vi "ImageListManager.vi"(8 "filename":string, 10 "Header Title String":string="Image List", 11 "Image Information In":T1) -> (3 "Image Information Out":T1)   [LabVIEW 2013]
uses:
  ImageInfoList.ctl
  <vilib>/Utility/sysdir.llb/System Directory Type.ctl
  <vilib>/Utility/xml.llb/Write to XML File(string).vi
  <vilib>/Utility/xml.llb/Read From XML File(string).vi
panel:
  out "Boolean References":refnum<vi>[](array[refnum])
  in  "Tab Control":enum32{"List", "Add"}(tab)
  in  "Image List":i32(listbox)
  in  "Add Button":bool
  in  "Remove Button":bool
  in  "Image Frequency (seconds)":dbl=30.0 min=30.0 step=1.0
  in  "Save Button":bool
  in  "Load Button":bool
  in  "Cancel Button":bool
  in  "OK Button":bool
  out "Help":string="This is the image management utility. \n\nTo add an image to the image list, click \"Add Image\" and you will be taken to the Add Image screen.  Provide a \"helpful name\" for the image either enter a file path to the image file or use the folder icon to browse.  You will be given a preview of your file.  To add the file to the list, press NEXT.  To exit the screen, press BACK.\n\nTo remove an image, select the image in the list and press \"Remove Image\".\n\nTo save your list of images, click \"Save List\".  To load your list of images for edit, click \"Load List\".  Lists will be saved in XML format.  Please do not edit the XML files directly.\n\nTo select the image frequency - or the amount of time between image updates, enter the Image Frequency into the box marked, \"Image Frequency (seconds)\".  \n\nTo accept this list of images, press OK.  To cancel all changes, press CANCEL."
  out "Error Messages":errorcluster
  out "Image Preview":picture
  in  "Back Button":bool
  in  "Next Button":bool
  in  "Image Path":path
  out "Add Image String":string="Add New Image"
  in  "Image Nickname":string
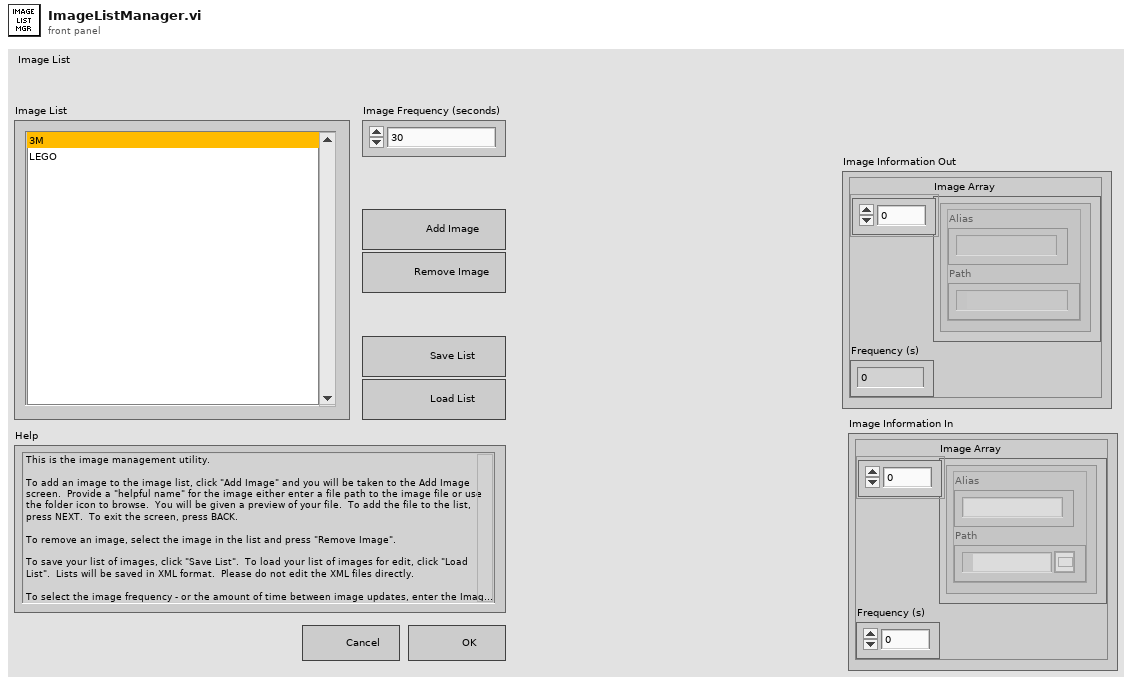
[diagram p1: front panel]
types:
  T1 = typedef "ImageInfoList.ctl" = cluster{"Image Array":cluster{"Alias":string, "Path":path}[], "Frequency (s)":dbl}
  T2 = enum8{"Enabled", "Disabled", "Disabled and Grayed Out"}
  T3 = typedef "System Directory Type.ctl" = i32
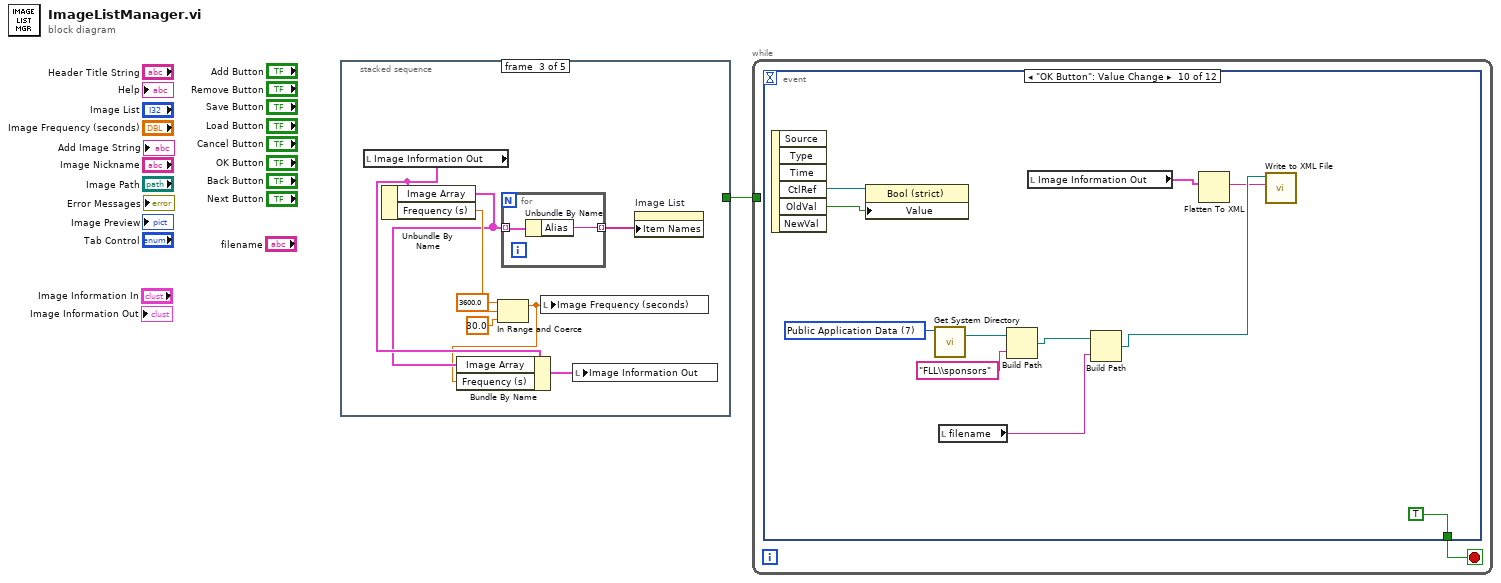
[diagram p0: block diagram]
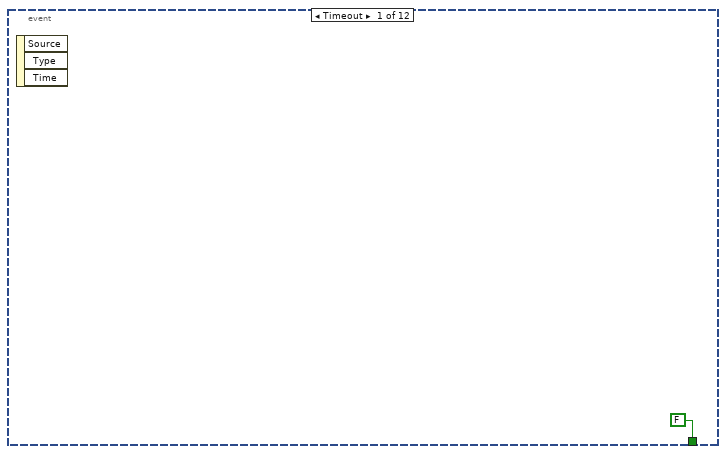
[diagram p2: hidden frame]
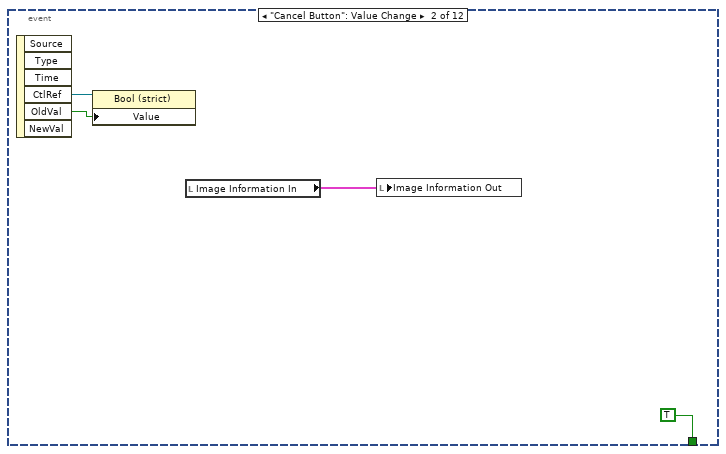
[diagram p3: hidden frame]
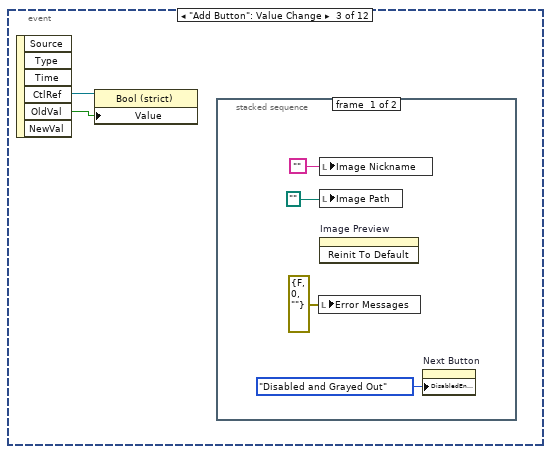
[diagram p4: hidden frame]
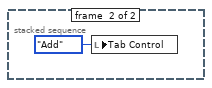
[diagram p5: hidden frame]
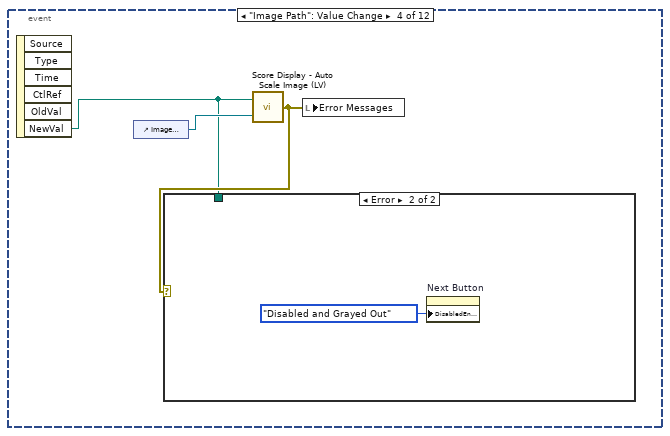
[diagram p6: hidden frame]
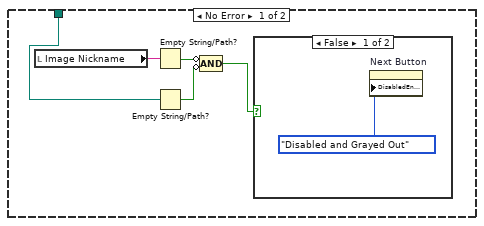
[diagram p7: hidden frame]
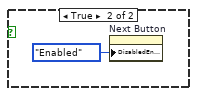
[diagram p8: hidden frame]
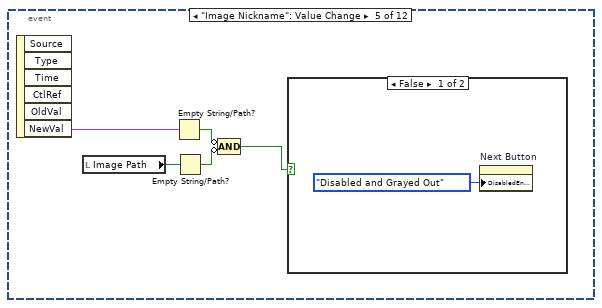
[diagram p9: hidden frame]
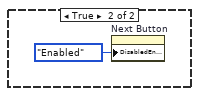
[diagram p10: hidden frame]
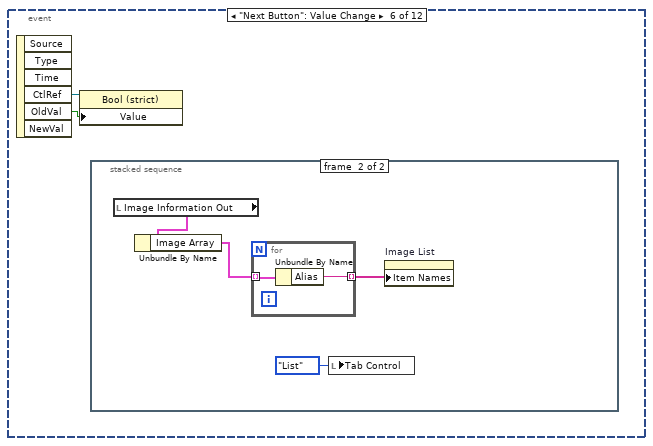
[diagram p11: hidden frame]
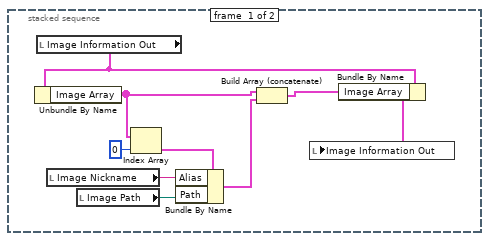
[diagram p12: hidden frame]
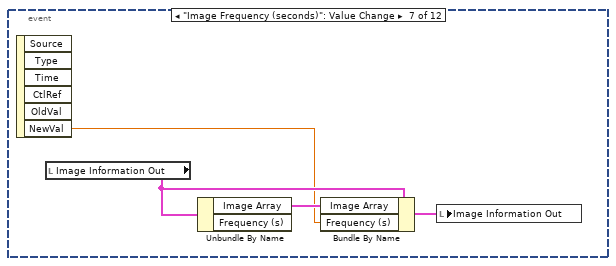
[diagram p13: hidden frame]
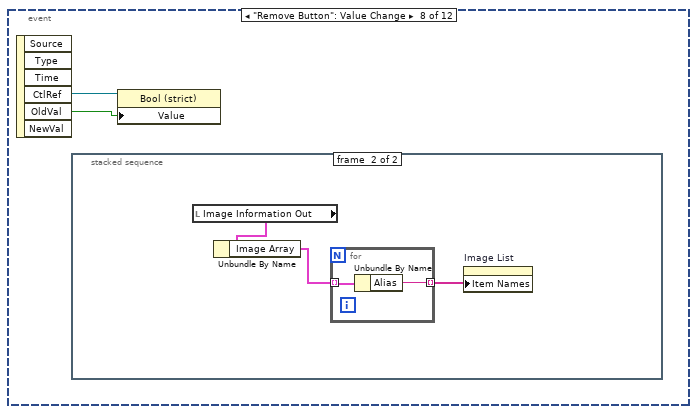
[diagram p14: hidden frame]
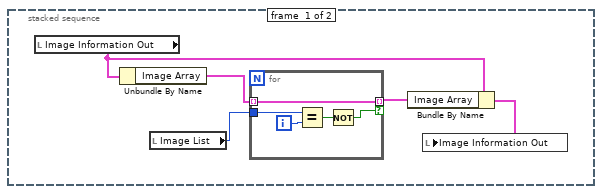
[diagram p15: hidden frame]
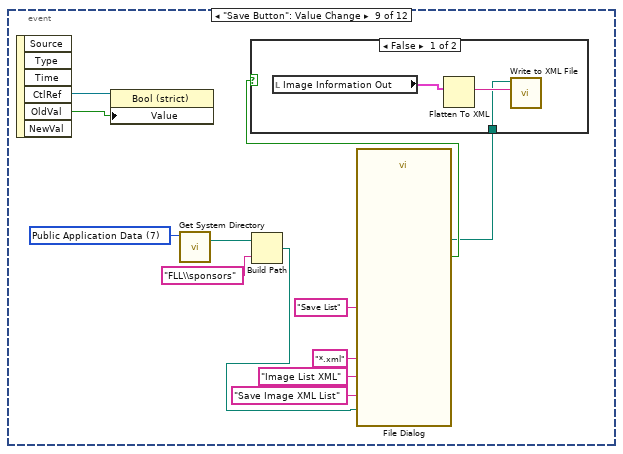
[diagram p16: hidden frame]
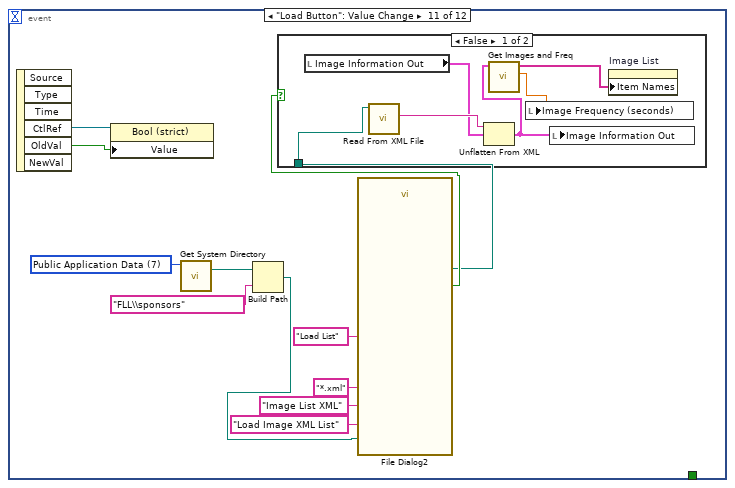
[diagram p18: hidden frame]
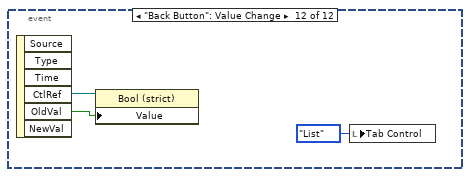
[diagram p20: hidden frame]
diagram:
  n1 = stacked-sequence {
    tunnel: [_ _ _ _ FALSE] -> w1
    frame #0 {
      n2 = control-ref of="Add Button"() -> (w2:refnum<vi>)
      n3 = control-ref of="Remove Button"() -> (w3:refnum<vi>)
      n4 = control-ref of="Save Button"() -> (w4:refnum<vi>)
      n5 = control-ref of="Load Button"() -> (w5:refnum<vi>)
      n6 = control-ref of="Cancel Button"() -> (w6:refnum<vi>)
      n7 = control-ref of="OK Button"() -> (w7:refnum<vi>)
      n8 = control-ref of="Back Button"() -> (w8:refnum<vi>)
      n9 = control-ref of="Next Button"() -> (w9:refnum<vi>)
      n10 = Build Array(w2, w3, w4, w5, w6, w7, w8, w9) -> (→"Boolean References":refnum<vi>[])
    }
    frame #1 {
      n11 = local read "Image Information In"() -> (w12:T1)
      n12 = local write "Tab Control"(enum32{"List", "Add"}."List" ("Tab Control")) -> ()
      n13 = local write "Image Information Out"(w12) -> ()
    }
    frame #2 {
      n14 = local read "Image Information Out"() -> (w15:T1)
      n15 = Unbundle By Name(w15) -> ("Image Array"=w14:cluster{"Alias":string, "Path":path}[], "Frequency (s)"=w19:dbl)
      n16 = In Range and Coerce(upper limit=3600.0, x=w19, lower limit=30.0) -> (coerced(x)=w13:dbl)  [unwired: 1 out]
      n17 = Bundle By Name(cluster=w15, "Image Array"=w14, "Frequency (s)"=w13) -> (w16:T1)
      n18 = for {
        tunnel: w14 -> [w22] mode=indexing
        tunnel: [w21] -> w20 mode=indexing
        n19 = Unbundle By Name(w22) -> ("Alias"=w21:string)
      }
      n20 = local write "Image Frequency (seconds)"(w13) -> ()
      n21 = local write "Image Information Out"(w16) -> ()
      n22 = property on="Image List" class="LstBox (strict)"("Item Names"=w20) -> ()  [unwired: 2 in, 2 out]
    }
    frame #3 {
      # "Initialize - Set Booleans to False"
      n23 = local read "Boolean References"() -> (w23:refnum<vi>[])
      n24 = for {
        tunnel: w23 -> [w25] mode=indexing
        n25 = property class="Bool (strict)"(reference=w25, "Value"=FALSE) -> ()  [unwired: 1 in, 2 out]
      }
    }
    frame #4 {
    }
  }
  n26 = while {
    tunnel: w1 -> [_]
    stop <- w27 stop-if-true
    n27 = event shown="[9] \"OK Button\": Value Change" {
      selector: _ -> [_ _ _ _ _ _ _ _ _ _ _ _]
      dyn-events: _ -> [_ _ _ _ _ _ _ _ _ _ _ _]
      timeout: _ -> [_ _ _ _ _ _ _ _ _ _ _ _]
      tunnel: [FALSE TRUE _ _ _ _ _ _ _ TRUE _ _] -> w27
      event Timeout {
        n28 = event-data() -> ()  [unwired: 1 in, 3 out]
      }
      event "Cancel Button": Value Change {
        n29 = event-data() -> ("CtlRef"=w30:refnum<vi>, "OldVal"=w29:bool)  [unwired: 1 in, 4 out]
        n30 = property class="Bool (strict)"(reference=w30, "Value"=w29) -> ()  [unwired: 1 in, 2 out]
        n31 = local read "Image Information In"() -> (w32:T1)
        n32 = local write "Image Information Out"(w32) -> ()
      }
      event "Add Button": Value Change {
        n33 = event-data() -> ("CtlRef"=w34:refnum<vi>, "OldVal"=w33:bool)  [unwired: 1 in, 4 out]
        n34 = property class="Bool (strict)"(reference=w34, "Value"=w33) -> ()  [unwired: 1 in, 2 out]
        n35 = stacked-sequence {
          frame #0 {
            n36 = local write "Error Messages"(errorcluster {"status"=FALSE, "code"=0, "source"=""} ("Error Messages")) -> ()
            n37 = local write "Image Nickname"("") -> ()
            n38 = local write "Image Path"(path "") -> ()
            n39 = invoke on="Image Preview" class="Pict" method="Reinit To Default"() -> ()  [unwired: 3 in, 3 out]
            n40 = property on="Next Button" class="Bool (strict)"("DisabledEnum"=T2."Disabled and Grayed Out" ("Disabled")) -> ()  [unwired: 2 in, 2 out]
          }
          frame #1 {
            n41 = local write "Tab Control"(enum32{"List", "Add"}."Add" ("Tab Control")) -> ()
          }
        }
      }
      event "Image Path": Value Change {
        n42 = event-data() -> ("NewVal"=w40:path)  [unwired: 1 in, 5 out]
        n43 = control-ref of="Image Preview"() -> (w42:refnum<vi>)
        n44 = call "Score Display - Auto Scale Image (LV).vi"("Picture Reference"=w42, "path to image file"=w40) -> ("error out"=w41:errorcluster)
        n45 = case shown="Error" w41 {
          tunnel: w40 -> [w45 _]
          frame No Error {
            n46 = local read "Image Nickname"() -> (w47:string)
            n47 = Empty String/Path?(string/path=w47) -> (empty?=w46:bool)
            n48 = Empty String/Path?(string/path=w45) -> (empty?=w44:bool)
            n49 = Compound Arithmetic op=AND(invert w46, invert w44) -> (w43:bool)
            n50 = case shown="False" w43 {
              frame False {
                n51 = property on="Next Button" class="Bool (strict)"("DisabledEnum"=T2."Disabled and Grayed Out" ("Disabled")) -> ()  [unwired: 2 in, 2 out]
              }
              frame True {
                n52 = property on="Next Button" class="Bool (strict)"("DisabledEnum"=T2."Enabled" ("Disabled")) -> ()  [unwired: 2 in, 2 out]
              }
            }
          }
          frame Error {
            n53 = property on="Next Button" class="Bool (strict)"("DisabledEnum"=T2."Disabled and Grayed Out" ("Disabled")) -> ()  [unwired: 2 in, 2 out]
          }
        }
        n54 = local write "Error Messages"(w41) -> ()
      }
      event "Image Nickname": Value Change {
        n55 = event-data() -> ("NewVal"=w55:string)  [unwired: 1 in, 5 out]
        n56 = local read "Image Path"() -> (w54:path)
        n57 = Empty String/Path?(string/path=w55) -> (empty?=w53:bool)
        n58 = Empty String/Path?(string/path=w54) -> (empty?=w52:bool)
        n59 = Compound Arithmetic op=AND(invert w53, invert w52) -> (w51:bool)
        n60 = case shown="False" w51 {
          frame False {
            n61 = property on="Next Button" class="Bool (strict)"("DisabledEnum"=T2."Disabled and Grayed Out" ("Disabled")) -> ()  [unwired: 2 in, 2 out]
          }
          frame True {
            n62 = property on="Next Button" class="Bool (strict)"("DisabledEnum"=T2."Enabled" ("Disabled")) -> ()  [unwired: 2 in, 2 out]
          }
        }
      }
      event "Next Button": Value Change {
        n63 = event-data() -> ("CtlRef"=w59:refnum<vi>, "OldVal"=w58:bool)  [unwired: 1 in, 4 out]
        n64 = property class="Bool (strict)"(reference=w59, "Value"=w58) -> ()  [unwired: 1 in, 2 out]
        n65 = stacked-sequence {
          frame #0 {
            n66 = local read "Image Information Out"() -> (w68:T1)
            n67 = Unbundle By Name(w68) -> ("Image Array"=w64:cluster{"Alias":string, "Path":path}[])
            n68 = local read "Image Nickname"() -> (w66:string)
            n69 = local read "Image Path"() -> (w65:path)
            n70 = Index Array(array=w64, index=0) -> (element=w67:cluster{"Alias":string, "Path":path})
            n71 = Bundle By Name(cluster=w67, "Alias"=w66, "Path"=w65) -> (w63:cluster{"Alias":string, "Path":path})
            n72 = Build Array (concatenate)(w64, w63) -> (w62:cluster{"Alias":string, "Path":path}[])
            n73 = Bundle By Name(cluster=w68, "Image Array"=w62) -> (w61:T1)
            n74 = local write "Image Information Out"(w61) -> ()
          }
          frame #1 {
            n75 = local read "Image Information Out"() -> (w71:T1)
            n76 = Unbundle By Name(w71) -> ("Image Array"=w70:cluster{"Alias":string, "Path":path}[])
            n77 = for {
              tunnel: w70 -> [w74] mode=indexing
              tunnel: [w73] -> w69 mode=indexing
              n78 = Unbundle By Name(w74) -> ("Alias"=w73:string)
            }
            n79 = local write "Tab Control"(enum32{"List", "Add"}."List" ("Tab Control")) -> ()
            n80 = property on="Image List" class="LstBox (strict)"("Item Names"=w69) -> ()  [unwired: 2 in, 2 out]
          }
        }
      }
      event "Image Frequency (seconds)": Value Change {
        n81 = event-data() -> ("NewVal"=w76:dbl)  [unwired: 1 in, 5 out]
        n82 = local read "Image Information Out"() -> (w78:T1)
        n83 = Unbundle By Name(w78) -> ("Image Array"=w77:cluster{"Alias":string, "Path":path}[])  [unwired: 1 out]
        n84 = Bundle By Name(cluster=w78, "Image Array"=w77, "Frequency (s)"=w76) -> (w75:T1)
        n85 = local write "Image Information Out"(w75) -> ()
      }
      event "Remove Button": Value Change {
        n86 = event-data() -> ("CtlRef"=w80:refnum<vi>, "OldVal"=w79:bool)  [unwired: 1 in, 4 out]
        n87 = stacked-sequence {
          frame #0 {
            n88 = local read "Image Information Out"() -> (w83:T1)
            n89 = Unbundle By Name(w83) -> ("Image Array"=w84:cluster{"Alias":string, "Path":path}[])
            n90 = local read "Image List"() -> (w85:i32)
            n91 = for {
              tunnel: w85 -> [w89]
              tunnel: w84 -> [w87] mode=indexing
              tunnel: [w87] -> w82 mode=indexing if=w86
              i -> [w90]
              n92 = Equal?(x=w89, y=w90) -> (x = y?=w88:bool)
              n93 = Not(x=w88) -> (.not. x?=w86:bool)
            }
            n94 = Bundle By Name(cluster=w83, "Image Array"=w82) -> (w81:T1)
            n95 = local write "Image Information Out"(w81) -> ()
          }
          frame #1 {
            n96 = local read "Image Information Out"() -> (w93:T1)
            n97 = Unbundle By Name(w93) -> ("Image Array"=w92:cluster{"Alias":string, "Path":path}[])
            n98 = for {
              tunnel: w92 -> [w95] mode=indexing
              tunnel: [w94] -> w91 mode=indexing
              n99 = Unbundle By Name(w95) -> ("Alias"=w94:string)
            }
            n100 = property on="Image List" class="LstBox (strict)"("Item Names"=w91) -> ()  [unwired: 2 in, 2 out]
          }
        }
        n101 = property class="Bool (strict)"(reference=w80, "Value"=w79) -> ()  [unwired: 1 in, 2 out]
      }
      event "Save Button": Value Change {
        w101 = T3 7 items=["User Home"=0, "User Desktop"=1, "User Documents"=2, "User Application Data"=3, "User Preferences"=4, "User Temporary"=5, "Public Documents"=6, "Public Application Data"=7, "Public Preferences"=8, "Public Cache"=13, "System Core Libraries"=9, "System Installed Libraries"=10, "Application Files"=11, "Boot Volume Root"=12] ("system directory type")
        n102 = event-data() -> ("CtlRef"=w107:refnum<vi>, "OldVal"=w106:bool)  [unwired: 1 in, 4 out]
        n103 = property class="Bool (strict)"(reference=w107, "Value"=w106) -> ()  [unwired: 1 in, 2 out]
        n104 = call <vilib>:"Get System Directory.vi"("system directory type"=w101) -> ("system directory"=w99:path)  [unwired: 10 in]
        n105 = Build Path(base path=w99, name or relative path="FLL\\sponsors") -> (appended path=w98:path)
        n106 = call "File Dialog"("start path"=w98, "prompt"="Save Image XML List", "button label"="Save List", "pattern (all files)"="*.xml", "pattern label"="Image List XML") -> ("selected path"=w96:path, "cancelled"=w97:bool)  [unwired: 7 in, 2 out]
        n107 = case shown="False" w97 {
          tunnel: w96 -> [w108 _]
          frame False {
            n108 = local read "Image Information Out"() -> (w110:T1)
            n109 = Flatten To XML(anything=w110) -> (xml string=w109:string)
            n110 = call-poly <vilib>:"Write to XML File.vi"("XML Input"=w109, "XML File Path"=w108) -> ()  [unwired: 7 in, 3 out]
          }
          frame True {
          }
        }
      }
      event "OK Button": Value Change {
        w119 = T3 7 items=["User Home"=0, "User Desktop"=1, "User Documents"=2, "User Application Data"=3, "User Preferences"=4, "User Temporary"=5, "Public Documents"=6, "Public Application Data"=7, "Public Preferences"=8, "Public Cache"=13, "System Core Libraries"=9, "System Installed Libraries"=10, "Application Files"=11, "Boot Volume Root"=12] ("system directory type")
        n111 = event-data() -> ("CtlRef"=w121:refnum<vi>, "OldVal"=w120:bool)  [unwired: 1 in, 4 out]
        n112 = property class="Bool (strict)"(reference=w121, "Value"=w120) -> ()  [unwired: 1 in, 2 out]
        n113 = call <vilib>:"Get System Directory.vi"("system directory type"=w119) -> ("system directory"=w117:path)  [unwired: 10 in]
        n114 = local read "filename"() -> (w115:string)
        n115 = Build Path(base path=w117, name or relative path="FLL\\sponsors") -> (appended path=w116:path)
        n116 = local read "Image Information Out"() -> (w113:T1)
        n117 = Build Path(base path=w116, name or relative path=w115) -> (appended path=w114:path)
        n118 = Flatten To XML(anything=w113) -> (xml string=w112:string)
        n119 = call-poly <vilib>:"Write to XML File.vi"("XML Input"=w112, "XML File Path"=w114) -> ()  [unwired: 7 in, 3 out]
      }
      event "Load Button": Value Change {
        w127 = T3 7 items=["User Home"=0, "User Desktop"=1, "User Documents"=2, "User Application Data"=3, "User Preferences"=4, "User Temporary"=5, "Public Documents"=6, "Public Application Data"=7, "Public Preferences"=8, "Public Cache"=13, "System Core Libraries"=9, "System Installed Libraries"=10, "Application Files"=11, "Boot Volume Root"=12] ("system directory type")
        n120 = event-data() -> ("CtlRef"=w133:refnum<vi>, "OldVal"=w132:bool)  [unwired: 1 in, 4 out]
        n121 = property class="Bool (strict)"(reference=w133, "Value"=w132) -> ()  [unwired: 1 in, 2 out]
        n122 = call <vilib>:"Get System Directory.vi"("system directory type"=w127) -> ("system directory"=w125:path)  [unwired: 10 in]
        n123 = Build Path(base path=w125, name or relative path="FLL\\sponsors") -> (appended path=w124:path)
        n124 = call "File Dialog2"("start path"=w124, "prompt"="Load Image XML List", "button label"="Load List", "pattern (all files)"="*.xml", "pattern label"="Image List XML") -> ("selected path"=w122:path, "cancelled"=w123:bool)  [unwired: 7 in, 2 out]
        n125 = case shown="False" w123 {
          tunnel: w122 -> [w137 _]
          frame False {
            n126 = local read "Image Information Out"() -> (w138:T1)
            n127 = call-poly <vilib>:"Read From XML File.vi"("XML File Path"=w137) -> ("XML Elements"=w139:string)  [unwired: 8 in, 2 out]
            n128 = Unflatten From XML(xml string=w139, type=w138) -> (value=w136:T1)  [unwired: 1 in, 1 out]
            n129 = call "Get Images and Freq.vi"("Image Information Out"=w136) -> ("upper limit"=w134:dbl, "Array"=w135:string[])  [unwired: 9 in]
            n130 = local write "Image Frequency (seconds)"(w134) -> ()
            n131 = local write "Image Information Out"(w136) -> ()
            n132 = property on="Image List" class="LstBox (strict)"("Item Names"=w135) -> ()  [unwired: 2 in, 2 out]
          }
          frame True {
          }
        }
      }
      event "Back Button": Value Change {
        n133 = event-data() -> ("CtlRef"=w141:refnum<vi>, "OldVal"=w140:bool)  [unwired: 1 in, 4 out]
        n134 = property class="Bool (strict)"(reference=w141, "Value"=w140) -> ()  [unwired: 1 in, 2 out]
        n135 = local write "Tab Control"(enum32{"List", "Add"}."List" ("Tab Control")) -> ()
      }
    }
  }
